vi "MBT_HandleReadError.vi"(8 "error in":errorcluster, 11 "ModbusExceptionCode":u8) -> (0 "error out":errorcluster, 3 "state":T1)   [LabVIEW 2012, in "MBT_ModbusTester.lvlib"]
uses:
  TSKMGR_TaskManager/mbTest_main_gui_states.ctl
  MBT_ModbusTester.lvlib
  TSKMGR_TaskManager/TSKMGR_TaskManager.lvlib
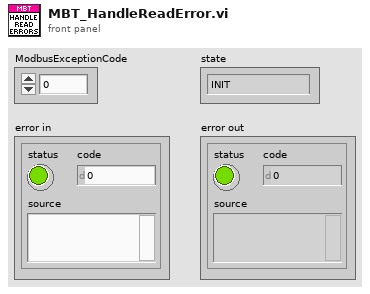
[diagram p1: front panel]
types:
  T1 = typedef "TSKMGR_TaskManager.lvlib/mbTest_main_gui_states.ctl" = enum16{"INIT", "IDLE", "CONNECT", "OPERATE", "DISCONNECT", "CLEAR", "EXIT_APP", "SAVE"}
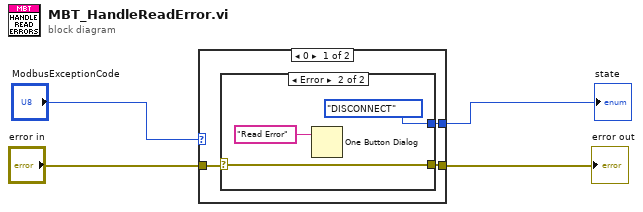
[diagram p0: block diagram]
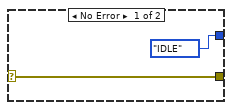
[diagram p2: hidden frame]
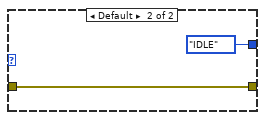
[diagram p3: hidden frame]
diagram:
  n1 = case shown="0" "ModbusExceptionCode" {
    tunnel: "error in" -> [w7 w14]
    tunnel: [w5 w14] -> w3
    tunnel: [w6 mbTest_main_gui_states."IDLE"] -> w4
    frame 0 {
      n2 = case shown="Error" w7 {
        selector: w7 -> [w8 w11]
        tunnel: [mbTest_main_gui_states."IDLE" mbTest_main_gui_states."DISCONNECT"] -> w6
        tunnel: [w8 w11] -> w5
        frame No Error {
        }
        frame Error {
          n3 = One Button Dialog(message="Read Error") -> ()  [unwired: 1 in, 1 out]
        }
      }
    }
    frame Default {
    }
  }
  "state" <- w4
  "error out" <- w3
